vi "format.timer.vi"(10 "dl timer":u32) -> (1 "seconds":dbl)   [LabVIEW 2024, in "Download_Manager.lvlib"]
uses:
  Download_Manager.lvlib
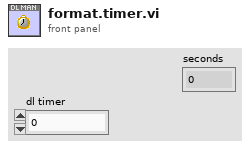
[diagram p1: front panel]
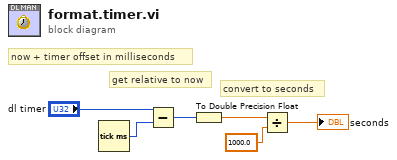
[diagram p0: block diagram]
diagram:
  # "convert to seconds"
  # "get relative to now"
  # "now + timer offset in milliseconds"
  n1 = Tick Count (ms)() -> (millisecond timer value=w4:u32)
  n2 = Subtract(x="dl timer", y=w4) -> (x-y=w6:u32)
  n3 = To Double Precision Float(number=w6) -> (double precision float=w2:dbl)
  n4 = Divide(x=w2, y=1000.0) -> (x/y=→"seconds":dbl)
